vi "Split Values Array.vi"(7 "#bytes per timestamp":i32, 9 "split index":i32, 10 "Values":u8[](array[numeric]), 11 "Timestamps":u64[](array[numeric])) -> (0 "Values (post-split)":u8[](array[numeric]), 1 "Timestamps (post-split)":u64[](array[numeric]), 2 "Values (pre-split)":u8[](array[numeric]), 3 "Timestamps (pre-split)":u64[](array[numeric]))   [LabVIEW 2021, in "Ring Buffer Time Series Data.lvlib"]
uses:
  Ring Buffer Time Series Data.lvlib
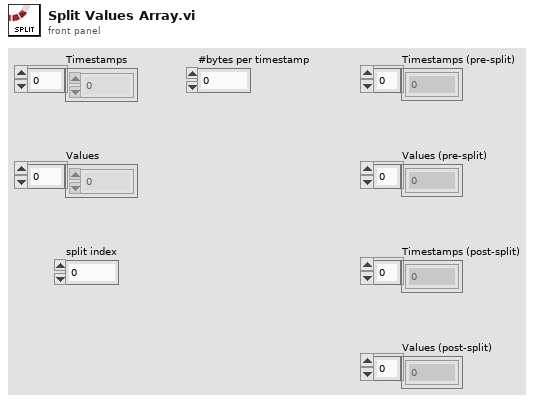
[diagram p1: front panel]
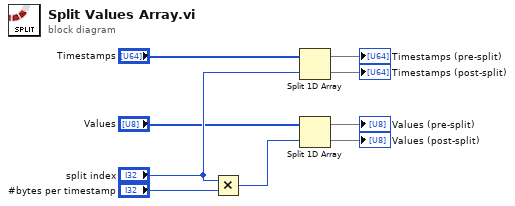
[diagram p0: block diagram]
diagram:
  n1 = Multiply(x="split index", y="#bytes per timestamp") -> (x*y=w5:i32)
  n2 = Split 1D Array(array="Timestamps", index="split index") -> (first subarray=→"Timestamps (pre-split)":u64[], second subarray=→"Timestamps (post-split)":u64[])
  n3 = Split 1D Array(array="Values", index=w5) -> (first subarray=→"Values (pre-split)":u8[], second subarray=→"Values (post-split)":u8[])
